vi "number1_sub1-login.vi"() -> (1 "UserCancelled":bool, 2 "Correct":bool)   [LabVIEW 2014]
panel:
  in  "Cancel":bool
  in  "Login":bool
  in  "Password":string
  in  "Username":string
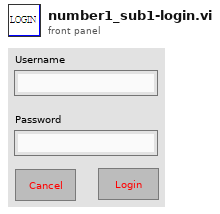
[diagram p1: front panel]
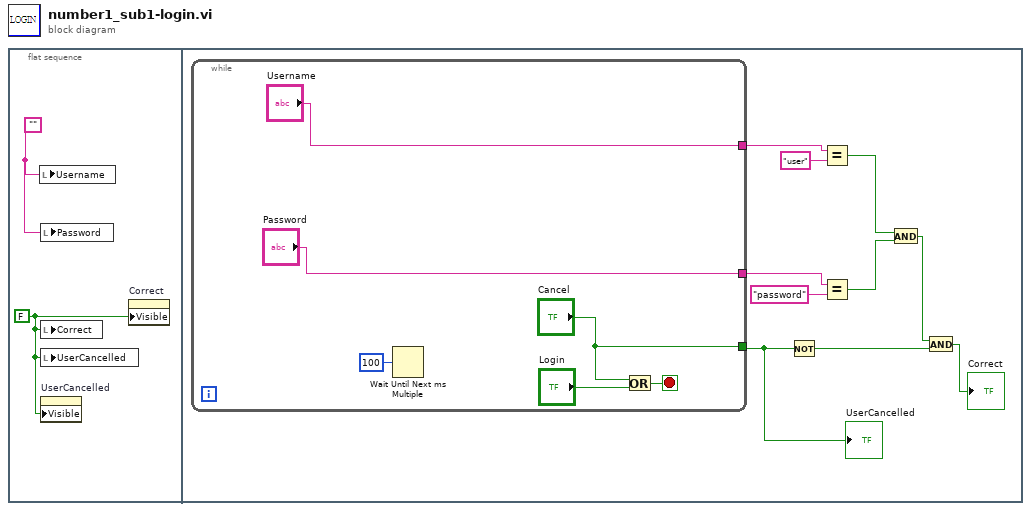
[diagram p0: block diagram]
diagram:
  n1 = flat-sequence {
    frame #0 {
      w1 = FALSE ("Correct")
      w2 = ""
      n2 = local write "Username"(w2) -> ()
      n3 = local write "Password"(w2) -> ()
      n4 = local write "Correct"(w1) -> ()
      n5 = local write "UserCancelled"(w1) -> ()
      n6 = property on="UserCancelled" class="Bool (strict)"("Visible"=w1) -> ()  [unwired: 2 in, 2 out]
      n7 = property on="Correct" class="Bool (strict)"("Visible"=w1) -> ()  [unwired: 2 in, 2 out]
    }
    frame #1 {
      n8 = while {
        tunnel: ["Username"] -> w8
        tunnel: ["Password"] -> w7
        tunnel: ["Cancel"] -> w3
        stop <- w15 stop-if-true
        n9 = Wait Until Next ms Multiple(millisecond multiple=u32 100) -> ()  [unwired: 1 out]
        n10 = Or(x="Cancel", y="Login") -> (x .or. y?=w15:bool)
      }
      "UserCancelled" <- w3
      n11 = Not(x=w3) -> (.not. x?=w5:bool)
      n12 = Equal?(x=w8, y="user") -> (x = y?=w11:bool)
      n13 = Equal?(x=w7, y="password") -> (x = y?=w12:bool)
      n14 = And(x=w11, y=w12) -> (x .and. y?=w4:bool)
      n15 = And(x=w4, y=w5) -> (x .and. y?=→"Correct":bool)
    }
  }
